vi "RunMethod.vi"(8 "error in (no error)":errorcluster caption="错误输入（无错误）", 9 "Data in":variant, 10 "vi reference":refnum<vi>, 11 "PanelLinkNode 输入":refnum<class "PanelLinkNode.lvclass"> caption="DNL_LabVIEW Object in") -> (0 "error out":errorcluster caption="错误输出", 1 "Data out":variant, 2 "vi reference out":refnum<vi>, 3 "PanelLinkNode 输出":refnum<class "PanelLinkNode.lvclass"> caption="DNL_LabVIEW Object out", 4 "Stop Traverse":bool)   [LabVIEW 2016, in "PanelLinkNode.lvclass"]
uses:
  PanelLinkNode.lvclass
panel:
  out "Method Name out":string
  in  "Method Name":string
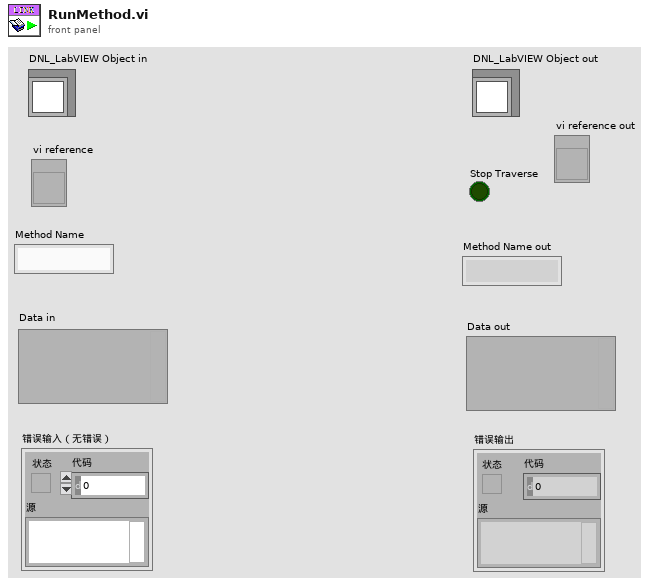
[diagram p1: front panel]
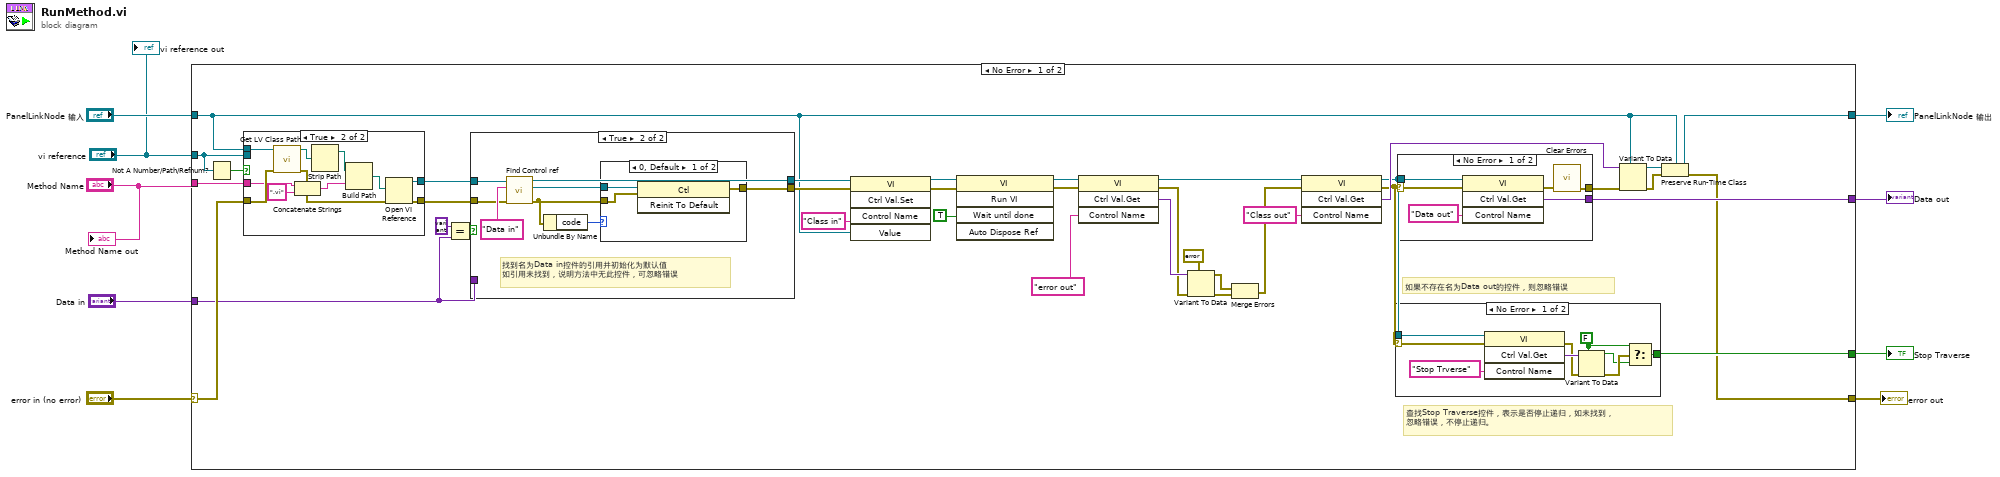
[diagram p0: block diagram]
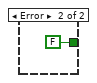
[diagram p3: hidden frame]
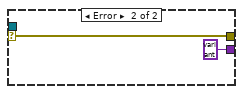
[diagram p4: hidden frame]
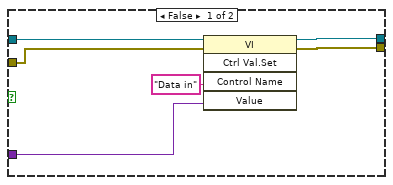
[diagram p5: hidden frame]
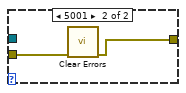
[diagram p6: hidden frame]
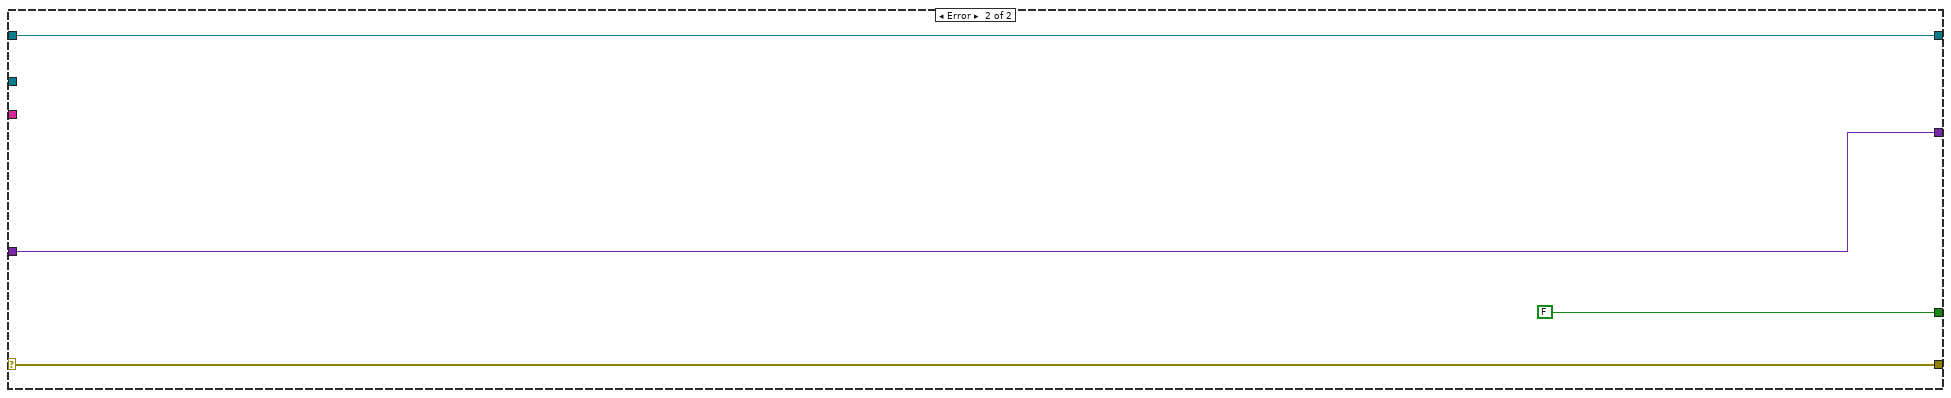
[diagram p7: hidden frame]
diagram:
  n1 = case shown="No Error" "error in (no error)" {
    selector: "error in (no error)" -> [w38 w100]
    tunnel: [w10 w100] -> w8
    tunnel: [w31 w99] -> w6
    tunnel: "PanelLinkNode 输入" -> [w33 w99]
    tunnel: "Data in" -> [w30 w97]
    tunnel: [w42 w97] -> w4
    tunnel: "Method Name" -> [w37 _]
    tunnel: [w25 FALSE] -> w3
    tunnel: "vi reference" -> [w21 _]
    frame No Error {
      # "查找Stop Traverse控件，表示是否停止递归，如未找到，\n忽略错误，不停止递归。"
      # "如果不存在名为Data out的控件，则忽略错误"
      n2 = Not A Number/Path/Refnum?(number/path/refnum=w21) -> (NaN/Path/Refnum?=w22:bool)
      n3 = case shown="True" w22 {
        tunnel: [w47 w57] -> w41
        tunnel: w38 -> [w47 w56]
        tunnel: w37 -> [_ w53]
        tunnel: w33 -> [_ w51]
        tunnel: [w48 w50] -> w23
        tunnel: w21 -> [w48 _]
        frame False {
        }
        frame True {
          n4 = call <vilib>:"Get LV Class Path.vi"("error in (no error)"=w56, "object"=w51) -> ("error out"=w55:errorcluster, "class path"=w59:path)  [unwired: 8 in]
          n5 = Concatenate Strings(w53, ".vi" ("字符串")) -> (w52:string)
          n6 = Strip Path(path=w59) -> (stripped path=w58:path)  [unwired: 1 out]
          n7 = Build Path(base path=w58, name or relative path=w52) -> (appended path=w49:path)
          n8 = Open VI Reference(vi path=w49, error in (no error)=w55) -> (vi reference=w50:refnum<vi>, error out=w57:errorcluster)  [unwired: 4 in]
        }
      }
      n9 = Equal?(x=variant, y=w30) -> (x = y?=w28:bool)
      n10 = case shown="True" w28 {
        tunnel: [w83 w89] -> w43
        tunnel: w23 -> [w82 w90]
        tunnel: w41 -> [w81 w86]
        tunnel: [w80 w88] -> w40
        tunnel: w30 -> [w78 _]
        frame False {
          n11 = invoke class="VI" method="Ctrl Val.Set"(reference=w82, error in=w81, "Control Name"="Data in" ("控件名"), "Value"=w78) -> (reference out=w83:refnum<vi>, error out=w80:errorcluster)  [unwired: 1 in, 3 out]
        }
        frame True {
          # "找到名为Data in控件的引用并初始化为默认值\n如引用未找到，说明方法中无此控件，可忽略错误"
          n12 = call "Find Control ref.vi"("error in (no error)"=w86, "control name"="Data in", "panelvi*"=w90) -> ("error out"=w84:errorcluster, "ctrl*"=w91:refnum<vi>, "panelvi* out"=w89:refnum<vi>)  [unwired: 6 in]
          n13 = Unbundle By Name(w84) -> ("code"=w85:i32)
          n14 = case shown="0, Default" w85 {
            tunnel: w91 -> [w94 _]
            tunnel: [w93 w95] -> w88
            tunnel: w84 -> [w92 w96]
            frame 0, Default {
              n15 = invoke class="Ctl" method="Reinit To Default"(reference=w94, error in=w92) -> (error out=w93:errorcluster)  [unwired: 1 in, 2 out]
            }
            frame 5001 {
              n16 = call <vilib>:"Clear Errors.vi"("error in (no error)"=w96) -> ("error out"=w95:errorcluster)  [unwired: 5 in, 1 out]
            }
          }
        }
      }
      n17 = invoke class="VI" method="Ctrl Val.Set"(reference=w43, error in=w40, "Control Name"="Class in" ("控件名"), "Value"=w33) -> (reference out=w45:refnum<vi>, error out=w39:errorcluster)  [unwired: 1 in, 3 out]
      n18 = invoke class="VI" method="Run VI"(reference=w45, error in=w39, "Wait until done"=TRUE ("结束前等待")) -> (reference out=w14:refnum<vi>, error out=w12:errorcluster)  [unwired: 2 in, 3 out]
      n19 = invoke class="VI" method="Ctrl Val.Get"(reference=w14, error in=w12, "Control Name"="error out" ("控件名")) -> (reference out=w13:refnum<vi>, error out=w17:errorcluster, "Get Control Value Variant"=w19:variant)  [unwired: 1 in, 1 out]
      n20 = Variant To Data(error in=w17, type=errorcluster {"status"=FALSE, "code"=0, "source"=""} ("错误输出"), Variant=w19) -> (data=w16:errorcluster, error out=w15:errorcluster)
      n21 = Merge Errors(w16, w15) -> (w11:errorcluster)
      n22 = invoke class="VI" method="Ctrl Val.Get"(reference=w13, error in=w11, "Control Name"="Class out" ("控件名")) -> (reference out=w26:refnum<vi>, error out=w24:errorcluster, "Get Control Value Variant"=w34:variant)  [unwired: 1 in, 1 out]
      n23 = case shown="No Error" w24 {
        selector: w24 -> [w66 _]
        tunnel: w26 -> [w67 _]
        tunnel: [w60 FALSE] -> w25
        frame No Error {
          w62 = FALSE
          n24 = invoke class="VI" method="Ctrl Val.Get"(reference=w67, error in=w66, "Control Name"="Stop Trverse" ("控件名")) -> (error out=w64:errorcluster, "Get Control Value Variant"=w65:variant)  [unwired: 1 in, 2 out]
          n25 = Variant To Data(error in=w64, type=w62, Variant=w65) -> (data=w61:bool, error out=w63:errorcluster)
          n26 = Select(t=w62, s=w63, f=w61) -> (s? t:f=w60:bool)
        }
        frame Error {
        }
      }
      n27 = case shown="No Error" w24 {
        selector: w24 -> [w72 w76]
        tunnel: [w74 variant ("Get Control Value Variant")] -> w42
        tunnel: w26 -> [w73 _]
        tunnel: [w70 w76] -> w27
        frame No Error {
          n28 = invoke class="VI" method="Ctrl Val.Get"(reference=w73, error in=w72, "Control Name"="Data out" ("控件名")) -> (error out=w71:errorcluster, "Get Control Value Variant"=w74:variant)  [unwired: 1 in, 2 out]
          n29 = call <vilib>:"Clear Errors.vi"("error in (no error)"=w71) -> ("error out"=w70:errorcluster)  [unwired: 5 in, 1 out]
        }
        frame Error {
        }
      }
      n30 = Variant To Data(error in=w27, type=w33, Variant=w34) -> (data=w36:refnum<class "PanelLinkNode.lvclass">, error out=w32:errorcluster)
      n31 = Preserve Run-Time Class(object in=w36, error in=w32, 2:w33) -> (object out=w31:refnum<class "PanelLinkNode.lvclass">, error out=w10:errorcluster)
    }
    frame Error {
    }
  }
  "error out" <- w8
  "PanelLinkNode 输出" <- w6
  "Data out" <- w4
  "Stop Traverse" <- w3
  "Method Name out" <- "Method Name"
  "vi reference out" <- "vi reference"
